vi "Reset.vi"(8 "error in (no error)":errorcluster, 11 "AbstractCollector2D in":refnum<class "AbstractCollector2D.lvclass">) -> (0 "error out":errorcluster, 3 "AbstractCollector2D out":refnum<class "AbstractCollector2D.lvclass">)   [LabVIEW 2014, in "AbstractCollector2D.lvclass"]
uses:
  AbstractCollector2D.lvclass
  Model/Data/Data2D/Data2D.lvclass
  AbstractCollector/AbstractCollector.lvclass
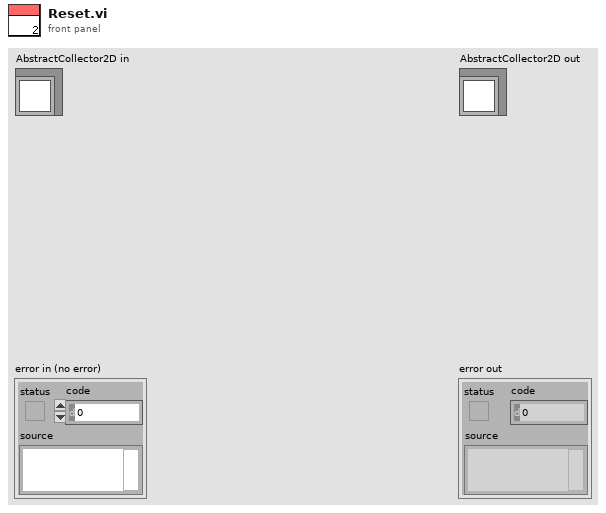
[diagram p1: front panel]
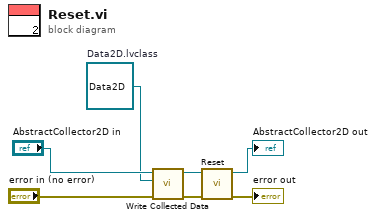
[diagram p0: block diagram]
diagram:
  w1 = refnum<class "Data2D.lvclass"> refnum  # Data2D.lvclass
  n1 = call-dynamic "Write Collected Data.vi"("error in (no error)"="error in (no error)", "Collected Data"=w1, "AbstractCollector in"="AbstractCollector2D in") -> ("error out"=w2:errorcluster, "AbstractCollector out"=w4:refnum<class "AbstractCollector2D.lvclass">)  [unwired: 7 in]
  n2 = call-parent "Reset.vi"("error in (no error)"=w2, "AbstractCollector in"=w4) -> ("error out"=→"error out":errorcluster, "AbstractCollector out"=→"AbstractCollector2D out":refnum<class "AbstractCollector2D.lvclass">)  [unwired: 8 in]
